vi "setFPGA.vi"(10 "FPGA":refnum<class "FPGA.lvclass">, 11 "TimestampControlFIFO in":refnum<class "TimestampControlFIFO.lvclass">) -> (3 "TimestampControlFIFO out":refnum<class "TimestampControlFIFO.lvclass">)   [LabVIEW 2016, in "TimestampControlFIFO.lvclass"]
uses:
  TimestampControlFIFO.lvclass
  FPGA/FPGA.lvclass
  TimestampControlFIFO.lvclass/TimestampControlFIFO.ctl
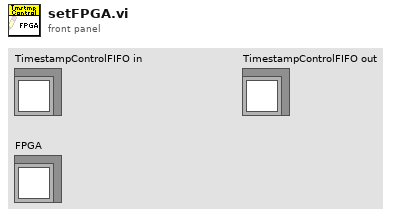
[diagram p1: front panel]
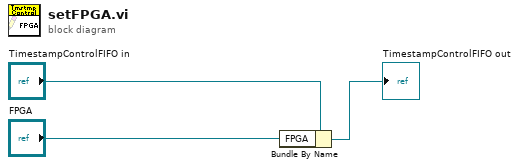
[diagram p0: block diagram]
diagram:
  n1 = Bundle By Name(cluster="TimestampControlFIFO in", "FPGA"="FPGA") -> (→"TimestampControlFIFO out":refnum<class "TimestampControlFIFO.lvclass">)
